vi "RunUnitTest.vi"(8 "error in (no error)":errorcluster) -> (0 "error out":errorcluster)   [LabVIEW 2020, in "CICD.lvlib"]
uses:
  CICD.lvlib
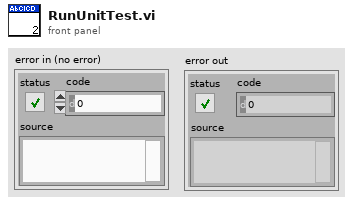
[diagram p1: front panel]
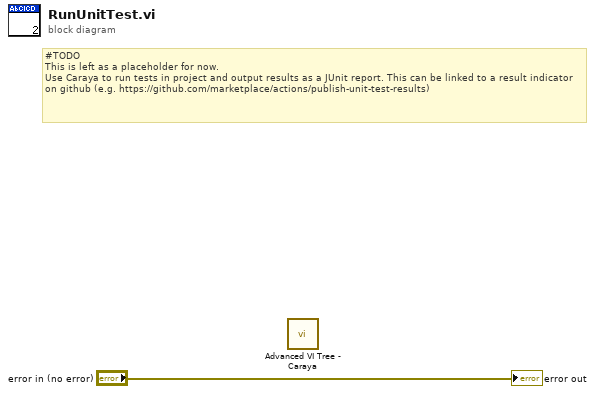
[diagram p0: block diagram]
diagram:
  # "#TODO\nThis is left as a placeholder for now.\nUse Caraya to run tests in project and output results as a JUnit report. This can be linked to a result indicator on github (e.g. https://github.com/marketplace/actions/publish-unit-test-results)"
  n1 = call <vilib>:"Advanced VI Tree - Caraya.vi"() -> ()  [unwired: 1 in]
  "error out" <- "error in (no error)"
